vi "Emballage_BDD_lecture_SNPROUIT_2D.vi"(8 "Error in":errorcluster caption="Error in (no error)", 11 "Famille":string) -> (0 "Error out":errorcluster, 1 "emplacement_autre":string, 2 "Fin_SNPRODUIT":string, 3 "Debut_SNPRODUIT":string, 4 "FIN_IDARTICLE":string, 5 "Debut_IDARTICLE":string)   [LabVIEW 2020]
uses:
  Modules/FS/60_FS_Controles/60_FS_SetGet.ctl
  <vilib>/drjdpowell/SQLite Library/SQL Connection/Open (path).vi
  <vilib>/drjdpowell/SQLite Library/SQL Connection/Open (string).vi
  <vilib>/AdvancedString/Path To Command Line String.vi
  <vilib>/drjdpowell/SQLite Library/SQL Connection/Connection.lvclass
panel:
  out "Column Names":string[](array[string])
  out "Result Set":string[][](table) caption="Result Set (from first statement with results)"
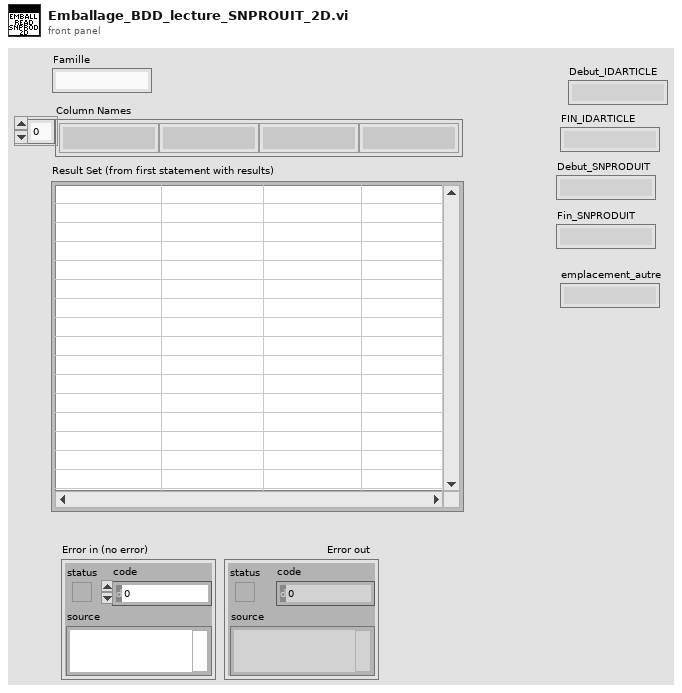
[diagram p1: front panel]
types:
  T1 = typedef "60_FS_SetGet.ctl" = enum16{"set", "get"}
  T2 = typedef "60_FS_CLT_Chemins.ctl" = cluster{"Racine_local":path, "Racine_reseau":path, "Racine_Support_Application":path, "Fichier_Journalisation":path, "Connexion_BDD_VSX":path, "Connexion_BDD_PLZ":path}
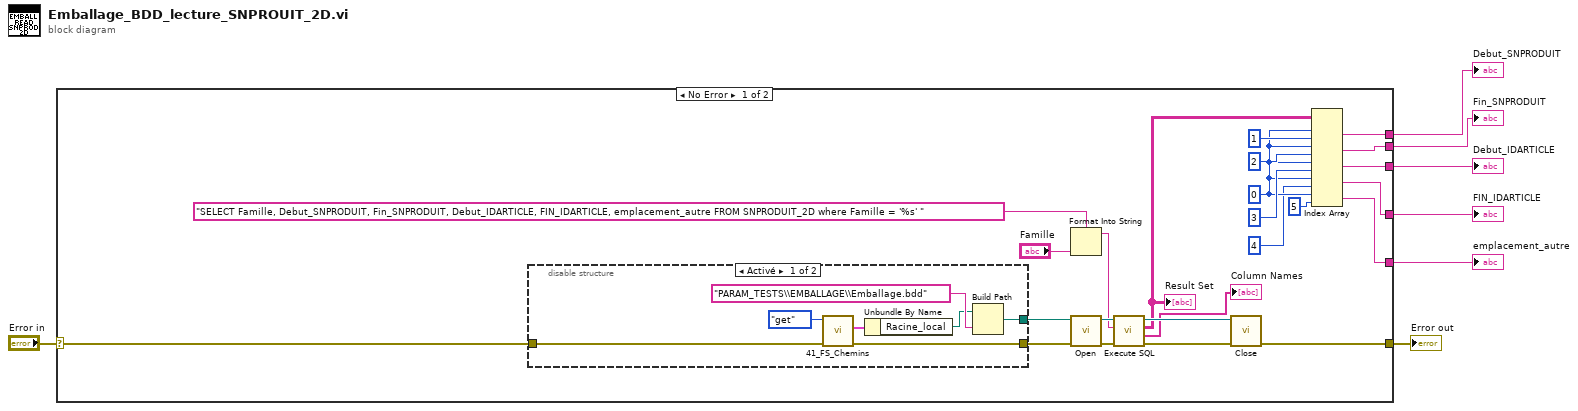
[diagram p0: block diagram]
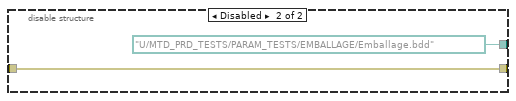
[diagram p2: hidden frame]
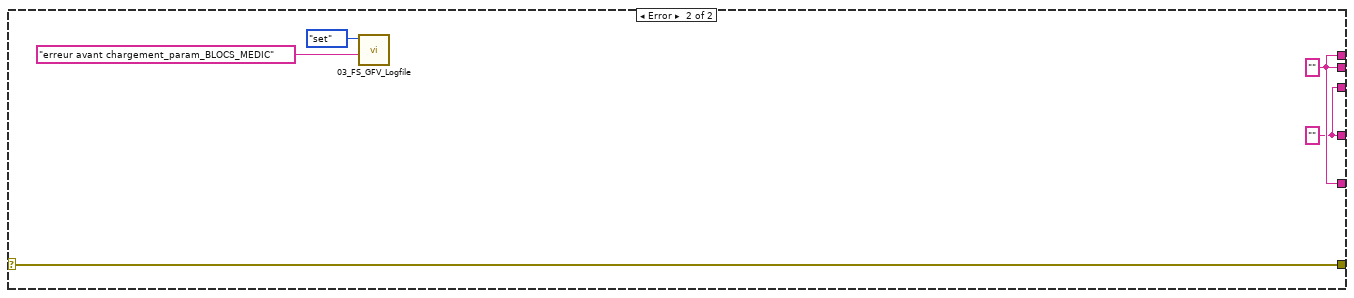
[diagram p3: hidden frame]
diagram:
  n1 = case shown="No Error" "Error in" {
    selector: "Error in" -> [w23 w45]
    tunnel: [w24 w45] -> w7
    tunnel: [w16 w42] -> w5
    tunnel: [w15 w42] -> w4
    tunnel: [w12 w42] -> w3
    tunnel: [w9 w41] -> w2
    tunnel: [w8 w41] -> w1
    frame No Error {
      w13 = 0 ("indice (ligne)")
      n2 = disable-structure shown="Activé" {
        disable-tunnel: [w36 path "U:/MTD_PRD_TESTS/PARAM_TESTS/EMBALLAGE/Emballage.bdd" ("appended path")] -> w31
        disable-tunnel: [w34 w40] -> w27
        disable-tunnel: w23 -> [w32 w40]
        frame Enabled {
          n3 = call "41_FS_Chemins.vi"("error in (no error)"=w32, "SetGet"=60_FS_SetGet."get") -> ("error out"=w34:errorcluster, "CLT_Chemins_out"=w33:T2)  [unwired: 8 in]
          n4 = Unbundle By Name(w33) -> ("Racine_local"=w37:path)
          n5 = Build Path(base path=w37, name or relative path="PARAM_TESTS\\EMBALLAGE\\Emballage.bdd" ("nom ou chemin relatif")) -> (appended path=w36:path)
        }
        frame Disabled {
        }
      }
      n6 = Format Into String(format string="SELECT Famille, Debut_SNPRODUIT, Fin_SNPRODUIT, Debut_IDARTICLE, FIN_IDARTICLE, emplacement_autre FROM SNPRODUIT_2D where Famille = '%s' " ("SQL"), "Famille") -> (resulting string=w21:string)  [unwired: 2 in, 1 out]
      n7 = call-poly <vilib>:"Open.vi"("error in (no error)"=w27, "db file"=w31) -> ("error out"=w25:errorcluster, "SQLite Connection"=w30:refnum<class "Connection.lvclass">)  [unwired: 8 in]
      n8 = call <vilib>:"Execute SQL.vi"("error in (no error)"=w25, "SQL"=w21, "SQLite Connection in"=w30) -> ("error out"=w28:errorcluster, "Column Names"=→"Column Names":string[], "Result Set"=w19:string[][], "SQLite Connection"=w29:refnum<class "Connection.lvclass">)  [unwired: 5 in]
      "Result Set" <- w19
      n9 = call-dynamic "Close.vi"("error in (no error)"=w28, "SQLite Connection in"=w29) -> ("error out"=w24:errorcluster)  [unwired: 9 in]
      n10 = Index Array(array=w19, index (row) #1=w13, index (col) #1=1 ("indice désactivé (col)"), index (row) #2=w13, index (col) #2=2 ("indice désactivé (col)"), index (row) #3=w13, index (col) #3=3 ("indice désactivé (col)"), index (row) #4=w13, index (col) #4=4 ("indice désactivé (col)"), index (row) #5=w13, index (col) #5=5 ("indice désactivé (col)")) -> (element #1=w16:string, element #2=w15:string, element #3=w9:string, element #4=w8:string, element #5=w12:string)
    }
    frame Error {
      w41 = ""
      w42 = ""
      n11 = call "03_FS_GFV_Logfile.vi"("Chaîne"="erreur avant chargement_param_BLOCS_MEDIC", "States"=60_FS_SetGet."set") -> ()  [unwired: 8 in, 2 out]
    }
  }
  "Error out" <- w7
  "Debut_SNPRODUIT" <- w5
  "Fin_SNPRODUIT" <- w4
  "emplacement_autre" <- w3
  "Debut_IDARTICLE" <- w2
  "FIN_IDARTICLE" <- w1
